vi "Pack Spectra.vi"(0 "magnitude spectra in":cluster{"f0":dbl, "df":dbl, "magnitude":dbl[]}[](array[cluster]), 4 "spectrum info":T1[](array[typedef]) {"x-axis units" items=["Time (s)"=0, "Frequency-CB (Hz)"=1, "Frequency-CPB (Hz)"=1248, "Frequency-Arbitrary (Hz)"=2357, "Quefrency (s)"=2, "Revolutions (rev)"=3, "Order"=4, "Speed (RPM)"=11, "Speed (rad/s)"=21, "Index"=65535]; "weighting filter" items=["Linear", "A-weighting", "B-weighting", "C-weighting", "ITU-R 468-4", "Dolby", "CCITT", "C-message", "Wb", "Wc", "Wd", "We", "Wf", "Wh", "Wj", "Wk", "Wm", "AES17 20 kHz lowpass", "AES17 40 kHz lowpass", "AES17 20 kHz highpass", "AES17 40 kHz highpass"]; "dB reference [EU]" format="%.2f"; "engineering units" items=["custom..."=0, "V"=1, "A"=21, "C"=30, "pC"=31, "s"=32, "-"=29, "Pa"=2, "N"=20, "g"=3, "m/s^2"=4, "m/s"=5, "m"=6, "mm/s"=12, "mm"=13, "micron/s"=14, "micron"=15, "in/s^2"=7, "in/s"=8, "in"=9, "mil/s"=10, "mil"=11, "rad/s^2"=16, "rad/s"=17, "rad"=18, "deg/s^2"=26, "deg/s"=27, "deg"=28, "RPM"=22, "cycle/s^2"=23, "Hz"=24, "cycle"=25, "strain"=19]; "spectral info"."window" items=["None "=0, "Hanning"=1, "Hamming"=2, "Blackman-Harris"=3, "Exact Blackman"=4, "Blackman"=5, "Flat Top"=6, "4 Term B-Harris "=7, "7 Term B-Harris"=8, "Low Sidelobe"=9, "Force - Exponential"=10, "Gaussian"=62]}) -> (14 "packed spectra":dbl[][](array[numeric]), 18 "spectra info":string[][](array[string]))   [LabVIEW 2024, in "Dynamic Signal Acquisition (Interactive).lvlib"]
uses:
  <vilib>/addons/_NISVFA/_Shared subVIs/Controls/svc_Spectrum Info.ctl
  <vilib>/addons/_NISVFA/_Shared subVIs/Controls/svc_X-Axis Units.ctl
  <vilib>/addons/_NISVFA/_Shared subVIs/Controls/svc_Spectrum Type.ctl
  <vilib>/addons/_NISVFA/_Shared subVIs/Controls/svc_Engineering Units Text Ring.ctl
  <vilib>/addons/_NISVFA/_Shared subVIs/Controls/svc_Weighting Filter Text Ring.ctl
  <vilib>/addons/_NISVFA/_Shared subVIs/Controls/svc_Complimentary Spectrum Units.ctl
  Dynamic Signal Acquisition (Interactive).lvlib
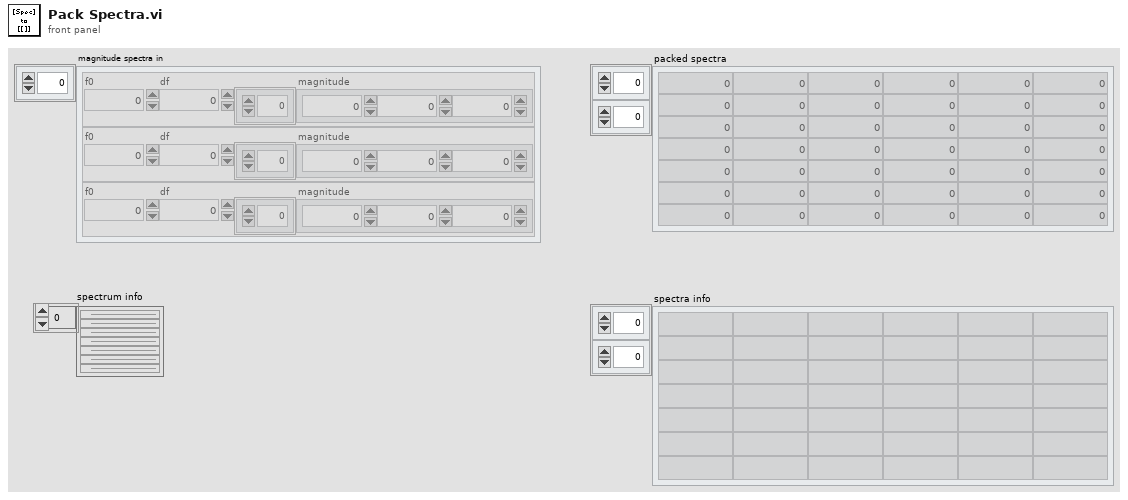
[diagram p1: front panel]
types:
  T1 = typedef "svc_Spectrum Info.ctl" = cluster{"channel name":string, "description":string, "x-axis units":T2, "spectral info":cluster{"spectrum type":T3, "linear/dB":enum16{"linear", "dB"}, "window":u16, "window size":i32, "FFT size":i32}, "engineering units":T4, "custom label":string, "dB reference [EU]":dbl, "peak units":enum16{"rms", "peak", "peak-peak"}, "weighting filter":T5, "spectral density?":bool, "unit label":string, "spectrum skewed?":bool, "complimentary spectrum units":T6}
  T2 = typedef "svc_X-Axis Units.ctl" = u16
  T3 = typedef "svc_Spectrum Type.ctl" = enum16{"FFT Spectrum [complex]", "Amplitude [Magnitude]", "Power [Magnitude^2]", "Cross Spectrum [complex]", "Frequency Response [Complex]"}
  T4 = typedef "svc_Engineering Units Text Ring.ctl" = u16
  T5 = typedef "svc_Weighting Filter Text Ring.ctl" = u16
  T6 = typedef "svc_Complimentary Spectrum Units.ctl" = enum16{"none", "radians", "degrees", "cycles", "imaginary"}
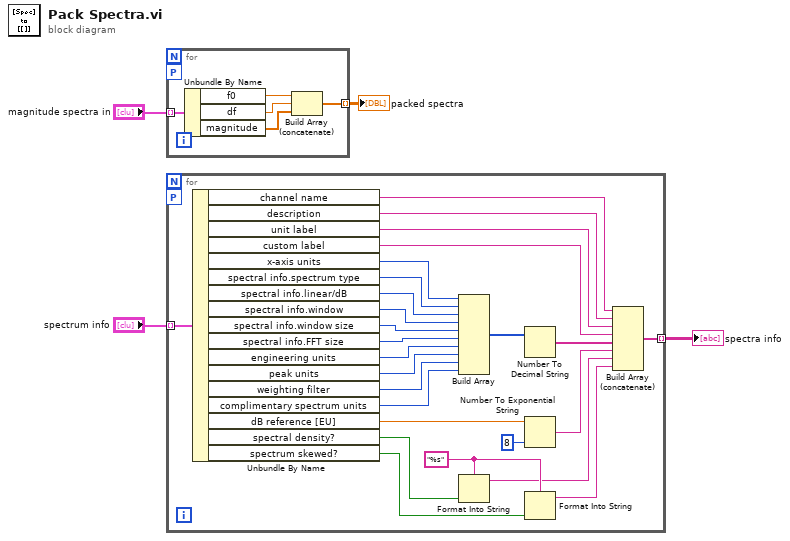
[diagram p0: block diagram]
diagram:
  n1 = for {
    tunnel: "magnitude spectra in" -> [w9] mode=indexing
    workers-P: _ -> [_]
    tunnel: [w5] -> w3 mode=indexing
    n2 = Unbundle By Name(w9) -> ("f0"=w8:dbl, "df"=w7:dbl, "magnitude"=w6:dbl[])
    n3 = Build Array (concatenate)(w8, w7, w6) -> (w5:dbl[])
  }
  "packed spectra" <- w3
  n4 = for {
    tunnel: "spectrum info" -> [w35] mode=indexing
    tunnel: [w10] -> w1 mode=indexing
    workers-P: _ -> [_]
    w16 = "%s" ("format string")
    n5 = Unbundle By Name(w35) -> ("channel name"=w21:string, "description"=w20:string, "unit label"=w19:string, "custom label"=w18:string, "x-axis units"=w32:T2, "spectral info.spectrum type"=w31:T3, "spectral info.linear/dB"=w30:enum16{"linear", "dB"}, "spectral info.window"=w29:u16, "spectral info.window size"=w28:i32, "spectral info.FFT size"=w27:i32, "engineering units"=w26:T4, "peak units"=w25:enum16{"rms", "peak", "peak-peak"}, "weighting filter"=w24:T5, "complimentary spectrum units"=w23:T6, "dB reference [EU]"=w34:dbl, "spectral density?"=w17:bool, "spectrum skewed?"=w15:bool)
    n6 = Build Array(w32, w31, w30, w29, w28, w27, w26, w25, w24, w23) -> (w22:i32[])
    n7 = Format Into String(format string=w16, w17) -> (resulting string=w12:string)  [unwired: 2 in, 1 out]
    n8 = Number To Decimal String(number=w22) -> (decimal integer string=w14:string[])  [unwired: 1 in]
    n9 = Number To Exponential String(number=w34, precision (6)=i16 8) -> (E-format string=w13:string)  [unwired: 2 in]
    n10 = Format Into String(format string=w16, w15) -> (resulting string=w11:string)  [unwired: 2 in, 1 out]
    n11 = Build Array (concatenate)(w21, w20, w19, w18, w14, w13, w12, w11) -> (w10:string[])
  }
  "spectra info" <- w1
